vi "LoadAdditionalData.vi"(8 "error in (no error)":errorcluster, 11 "TesteractHAL_DigitalOutput_EthernetModbus In":refnum<class "TesteractHAL_DigitalOutput_EthernetModbus.lvclass">) -> (0 "error out":errorcluster, 3 "TesteractHAL_DigitalOutput_EthernetModbus Out":refnum<class "TesteractHAL_DigitalOutput_EthernetModbus.lvclass">)   [LabVIEW 2017, in "TesteractHAL_DigitalOutput_EthernetModbus.lvlib" / "TesteractHAL_DigitalOutput_EthernetModbus.lvclass"]
uses:
  TesteractHAL_DigitalOutput_EthernetModbus.lvclass
  C:/Program Files (x86)/Testeract/HWLib/HAL/Device/TesteractHAL_Device.lvlibp/TesteractHAL_Device.lvclass
  TesteractHAL_DigitalOutput_EthernetModbus.lvclass/TesteractHAL_DigitalOutput_EthernetModbus.ctl
  Program Files (x86)/Testeract/HWLib/HAL/Device/TesteractHAL_Device.lvlibp/ReadDeviceName.vi
  Program Files (x86)/Testeract/HWLib/HAL/DeviceCfg/TesteractHAL_DeviceCfg_API.lvlibp
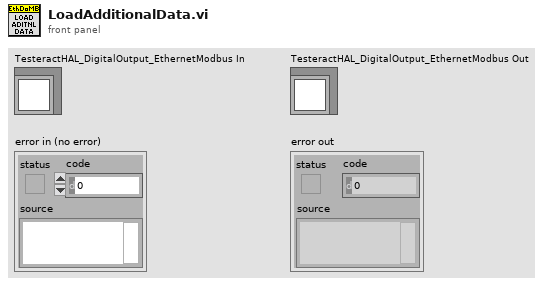
[diagram p1: front panel]
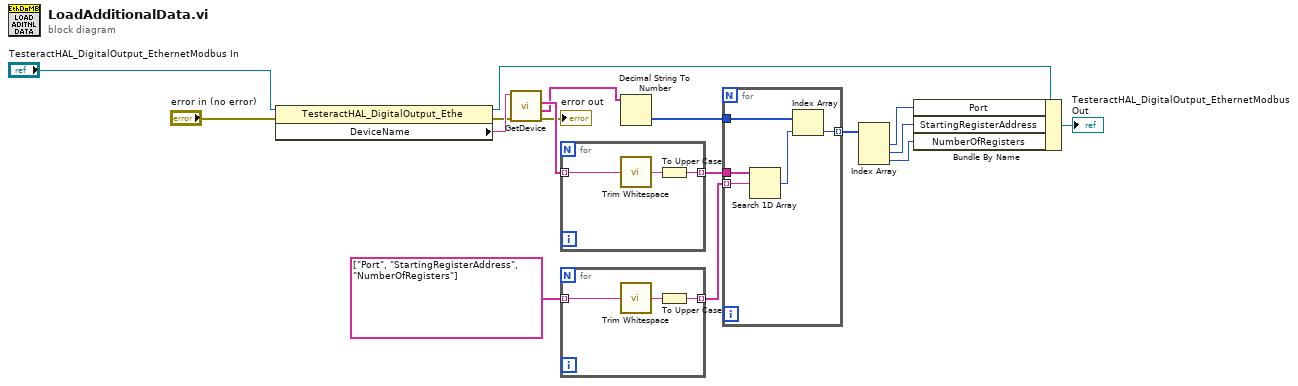
[diagram p0: block diagram]
diagram:
  n1 = property class="TesteractHAL_DigitalOutput_Ethe"(reference="TesteractHAL_DigitalOutput_EthernetModbus In", error in="error in (no error)") -> (reference out=w9:refnum<class "TesteractHAL_DigitalOutput_EthernetModbus.lvclass">, error out=w15:errorcluster, "DeviceName"=w16:string)
  n2 = call "GetDevice.vi"("error in (no error)"=w15, "Device"=w16) -> ("error out"=→"error out":errorcluster, "Values"=w14:string[], "Keys"=w17:string[])  [unwired: 6 in, 1 out]
  n3 = for {
    tunnel: w17 -> [w19] mode=indexing
    tunnel: [w18] -> w10 mode=indexing
    n4 = call <vilib>:"Trim Whitespace.vi"("string"=w19) -> ("trimmed string"=w20:string)  [unwired: 1 in]
    n5 = To Upper Case(1:w20) -> (0:w18:string)
  }
  n6 = for {
    tunnel: string[] ["Port", "StartingRegisterAddress", "NumberOfRegisters"] -> [w23] mode=indexing
    tunnel: [w21] -> w12 mode=indexing
    n7 = call <vilib>:"Trim Whitespace.vi"("string"=w23) -> ("trimmed string"=w22:string)  [unwired: 1 in]
    n8 = To Upper Case(1:w22) -> (0:w21:string)
  }
  n9 = Decimal String To Number(string=w14) -> (number=w11:i32[])  [unwired: 2 in, 1 out]
  n10 = for {
    tunnel: w10 -> [w28]
    tunnel: w12 -> [w27] mode=indexing
    tunnel: w11 -> [w25]
    tunnel: [w24] -> w8 mode=indexing
    n11 = Search 1D Array(1D array=w28, element=w27) -> (index of element=w26:i32)  [unwired: 1 in]
    n12 = Index Array(array=w25, index=w26) -> (element=w24:i32)
  }
  n13 = Index Array(array=w8) -> (element #1=w7:i32, element #2=w6:i32, element #3=w5:i32)  [unwired: 3 in]
  n14 = Bundle By Name(cluster=w9, "Port"=w7, "StartingRegisterAddress"=w6, "NumberOfRegisters"=w5) -> (→"TesteractHAL_DigitalOutput_EthernetModbus Out":refnum<class "TesteractHAL_DigitalOutput_EthernetModbus.lvclass">)
